vi "test_LoadHwXML.vi"() -> ()   [LabVIEW 2020]
uses:
  <instrlib>/BTICardLib/Private/Initialize By Card Number and Core Number.vi
  <instrlib>/BTI1553Lib/Private/Channel/Configure/Configure All From XML.vi
  <instrlib>/BTICardLib/BTICardLV.lvlib
  <instrlib>/BTI1553Lib/BTI1553LV.lvlib
  <instrlib>/BTICardLib/Private/Configure All From XML.vi
panel:
  out "channel count out":i32
  in  "channel handle array size in":i32
  out "XML load time ms":u32
  in  "card number":i32
  in  "core number":i32
  in  "configuration file path":path=path "c:/ni-rt/VeriStand/Custom Devices/Ballard - 1553/Board_1__Core_0__.xml"
  out "error out":errorcluster
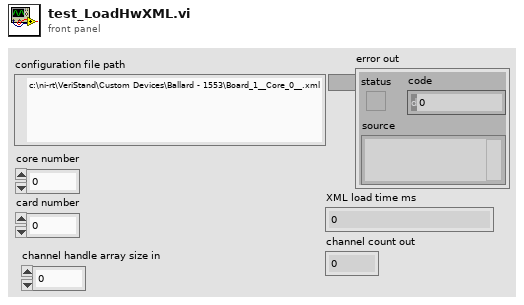
[diagram p1: front panel]
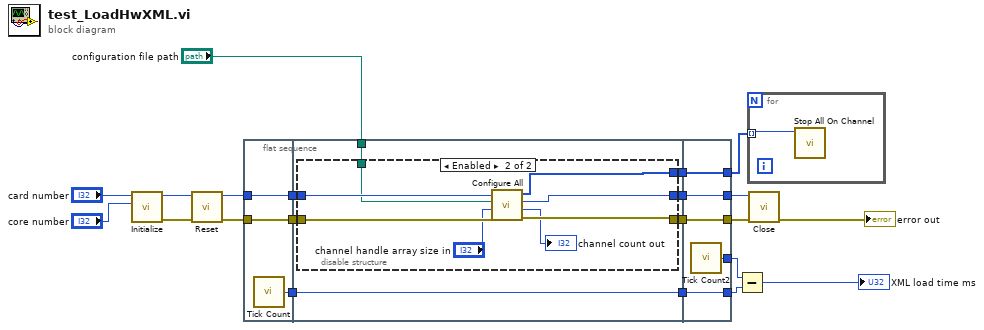
[diagram p0: block diagram]
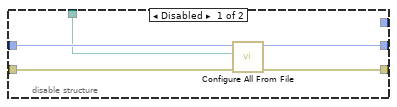
[diagram p2: hidden frame]
diagram:
  n1 = call-poly <instrlib>:"Initialize.vi"("core number"="core number", "card number"="card number") -> ("error out"=w19:errorcluster, "core handle out"=w18:u64)  [unwired: 8 in]
  n2 = call <instrlib>:"Reset.vi"("error in (no error)"=w19, "core handle in"=w18) -> ("error out"=w20:errorcluster, "core handle out"=w21:u64)  [unwired: 8 in]
  n3 = flat-sequence {
    tunnel: w20 -> [w23]
    tunnel: w21 -> [w24]
    tunnel: [w24] -> w10
    tunnel: [w23] -> w9
    tunnel: [w22] -> w5
    tunnel: [w29] -> w12
    tunnel: [w28] -> w11
    tunnel: w10 -> [w31]
    tunnel: w9 -> [w30]
    tunnel: [w27] -> w6
    tunnel: w5 -> [w27]
    tunnel: "configuration file path" -> [w26]
    tunnel: [w25] -> w2
    tunnel: [w48] -> w16
    tunnel: [w49] -> w17
    tunnel: w12 -> [w49]
    tunnel: w11 -> [w48]
    tunnel: [w47] -> w8
    tunnel: [w46] -> w7
    tunnel: w6 -> [w46]
    tunnel: [w45] -> w1
    tunnel: w2 -> [w45]
    frame #0 {
      n4 = call "Tick Count"() -> ("Tick Count(mSec)"=w22:u32)
    }
    frame #1 {
      n5 = disable-structure shown="Enabled" {
        disable-tunnel: w31 -> [w36 w44]
        disable-tunnel: w30 -> [w35 w43]
        disable-tunnel: [w34 w40] -> w29
        disable-tunnel: [w33 w39] -> w28
        disable-tunnel: w26 -> [w32 w41]
        disable-tunnel: [_ w37] -> w25
        frame Disabled {
          n6 = call-poly <instrlib>:"Configure All From File.vi"("error in (no error)"=w35, "configuration file path"=w32, "core handle in"=w36) -> ("error out"=w33:errorcluster, "core handle out"=w34:u64)  [unwired: 7 in]
        }
        frame Enabled {
          n7 = call-poly <instrlib>:"Configure All.vi"("error in (no error)"=w43, "channel handle array size in"="channel handle array size in", "configuration file path"=w41, "core handle in"=w44) -> ("error out"=w39:errorcluster, "channel count out"=→"channel count out":i32, "core handle out"=w40:u64, "channel handles out"=w37:u64[])  [unwired: 4 in]
        }
      }
    }
    frame #2 {
      n8 = call "Tick Count2"() -> ("Tick Count(mSec)"=w47:u32)
    }
  }
  n9 = Subtract(x=w8, y=w7) -> (x-y=→"XML load time ms":u32)
  n10 = for {
    tunnel: w1 -> [w50] mode=indexing
    n11 = call <instrlib>:"Stop All On Channel.vi"("channel handle in"=w50) -> ()  [unwired: 9 in, 2 out]
  }
  n12 = call <instrlib>:"Close.vi"("error in (no error)"=w16, "core handle in"=w17) -> ("error out"=→"error out":errorcluster)  [unwired: 8 in, 1 out]
